vi "Create Pattern Script - Rd Data Frame.vi"(8 "error in (no error)":errorcluster, 10 "FRM Data":T1 {"Addr" format="%x"; "Data" format="%x"}, 11 "SPI 3W Pattern Creator in":refnum<class "SPI 3W Pattern Creator.lvclass">) -> (0 "error out":errorcluster, 2 "String":string, 3 "SPI 3W Pattern Creator out":refnum<class "SPI 3W Pattern Creator.lvclass">)   [LabVIEW 2018, in "SPI 3W Pattern Creator.lvlib" / "SPI 3W Pattern Creator.lvclass"]
uses:
  SPI 3W Pattern Creator.lvclass
  Ctls/Frame Data - SPI_3W.ctl
  Ctls/RW Options.ctl
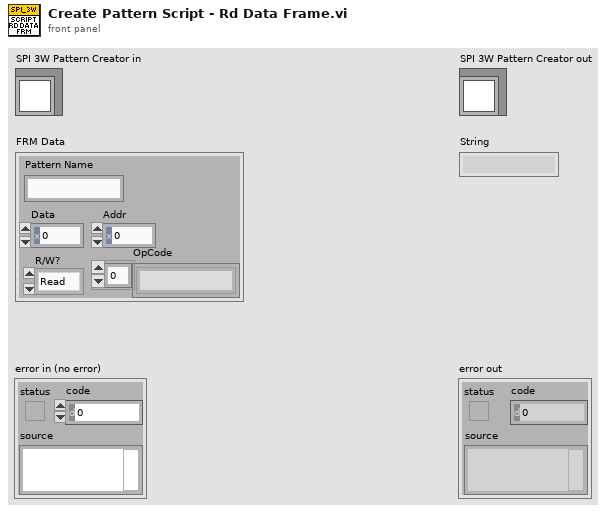
[diagram p1: front panel]
types:
  T1 = typedef "Frame Data - SPI_3W.ctl" = cluster{"Pattern Name":string, "Data":u16, "Addr":u16, "OpCode":string[], "R/W?":T2}
  T2 = typedef "RW Options.ctl" = enum16{"Read", "Write", "R/W"}
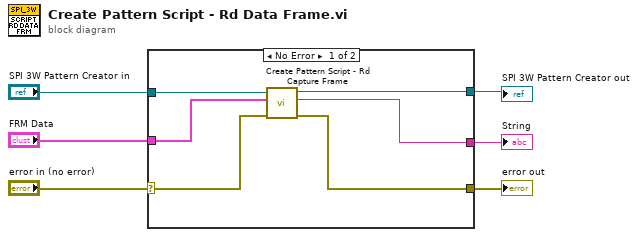
[diagram p0: block diagram]
diagram:
  n1 = case shown="No Error" "error in (no error)" {
    selector: "error in (no error)" -> [w10 w13]
    tunnel: "SPI 3W Pattern Creator in" -> [w12 w14]
    tunnel: "FRM Data" -> [w11 _]
    tunnel: [w9 w13] -> w3
    tunnel: [w8 w14] -> w2
    tunnel: [w7 _] -> w1
    frame No Error {
      n2 = call-dynamic "Create Pattern Script - Rd Capture Frame.vi"("error in (no error)"=w10, "FRM Data"=w11, "SPI 3W Pattern Creator in"=w12) -> ("error out"=w9:errorcluster, "String"=w7:string, "SPI 3W Pattern Creator out"=w8:refnum<class "SPI 3W Pattern Creator.lvclass">)  [unwired: 6 in]
    }
    frame Error {
    }
  }
  "error out" <- w3
  "SPI 3W Pattern Creator out" <- w2
  "String" <- w1
